vi "ActionVIOnLoad.vi"(8 "error in (no error)":errorcluster, 11 "Device Item Ref in":T1 format="%.0x") -> (0 "error out":errorcluster, 3 "Device Item Ref out":T1 format="%.0x")   [LabVIEW 2015, in "J1939 Addon System Explorer.lvlib"]
uses:
  J1939 Addon System Explorer.lvlib
  <vilib>/NI Veristand/Custom Device API/Custom Device Item Ref.ctl
  Shared/Types/XNET Settings.ctl
  Shared/Types/Monitor Settings.ctl
  Shared/Types/SPN Properties.ctl
  NationalInstruments.VeriStand.SystemDefinitionAPI
  Shared/SubVIs/Constants.vi
  <vilib>/NI Veristand/Custom Device API/Get Item Property (Variant).vi
  <vilib>/NI Veristand/Custom Device Tools/Custom Device Utility Library/NI VeriStand - Search for Item by GUID.vi
  <vilib>/NI Veristand/Custom Device API/Get Item Property (U16).vi
  <vilib>/NI Veristand/Custom Device API/Set Item Property (String).vi
  <vilib>/NI Veristand/Custom Device Tools/Custom Device Utility Library/NI VeriStand - Search for All Items by GUID.vi
  <vilib>/NI VeriStand/Custom Device API/Custom Device API.lvlib
  Shared/J1939 Addon Shared.lvlib
  <vilib>/NI VeriStand/Custom Device Tools/Custom Device Utility Library/Custom Device Utility Library.lvlib
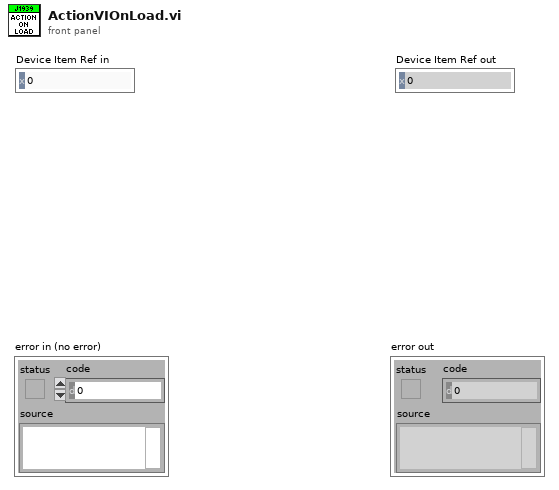
[diagram p1: front panel]
types:
  T1 = typedef "Custom Device API.lvlib/Custom Device Item Ref.ctl" = u64
  T2 = typedef "J1939 Addon Shared.lvlib/Monitor Settings.ctl" = cluster{"Address":u8, "Name":u64, "Include DA":bool}
  T3 = typedef "J1939 Addon Shared.lvlib/XNET Settings.ctl" = cluster{"Database":refnum<k21>, "Cluster":refnum<k21>, "Port":string, "Baud rate [Bd]":u32, "Termination":u32, "Incoming Decimation":u32, "Outgoing Decimation":u32}
  T4 = cluster{"XNET Database":refnum<k21>, "XNET Cluster":refnum<k21>, "CAN Port":string, "Baud rate [Bd]":u32, "J1939 Network Address":u8, "Name":u64, "Termination":u32}
  T5 = cluster{"XNET Database":refnum<k21>, "XNET Cluster":refnum<k21>, "CAN Port":string, "Baud rate [Bd]":u32, "J1939 Network Address":u8, "Name":u64, "Termination":u32, "Incoming Rate":u32, "Outcoming Rate":u32}
  T6 = cluster{"Database":refnum<k21>, "Cluster":refnum<k21>, "Port":string, "Baud rate [Bd]":u32, "Termination":u32, "Incoming Rate":u32, "Outcoming Rate":u32, "Write Decimation":u32}
  T7 = typedef "J1939 Addon Shared.lvlib/SPN Properties.ctl" = cluster{"Bytes":u32, "ScaleFac":dbl, "ScaleOff":dbl}
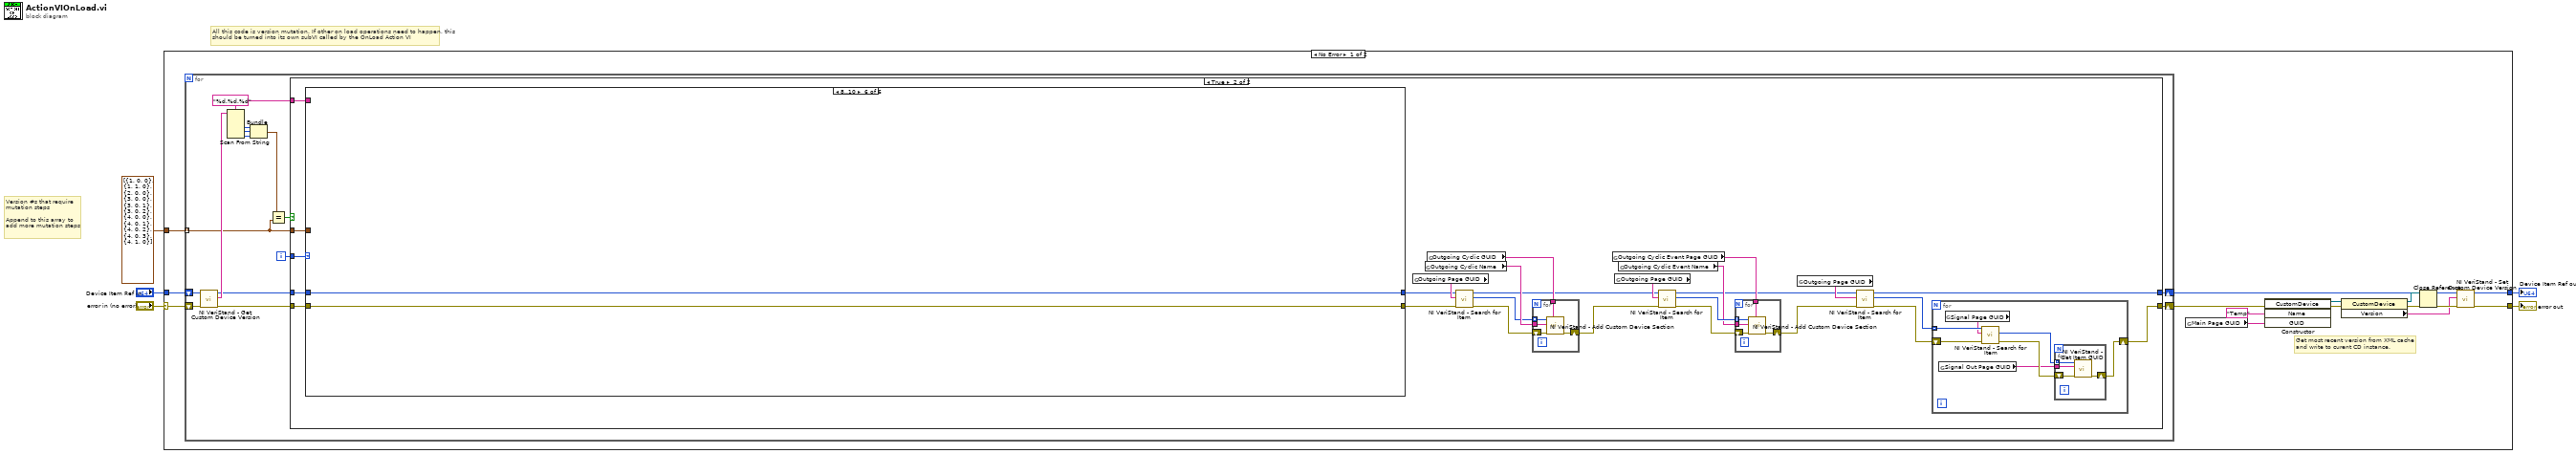
[diagram p0: block diagram]
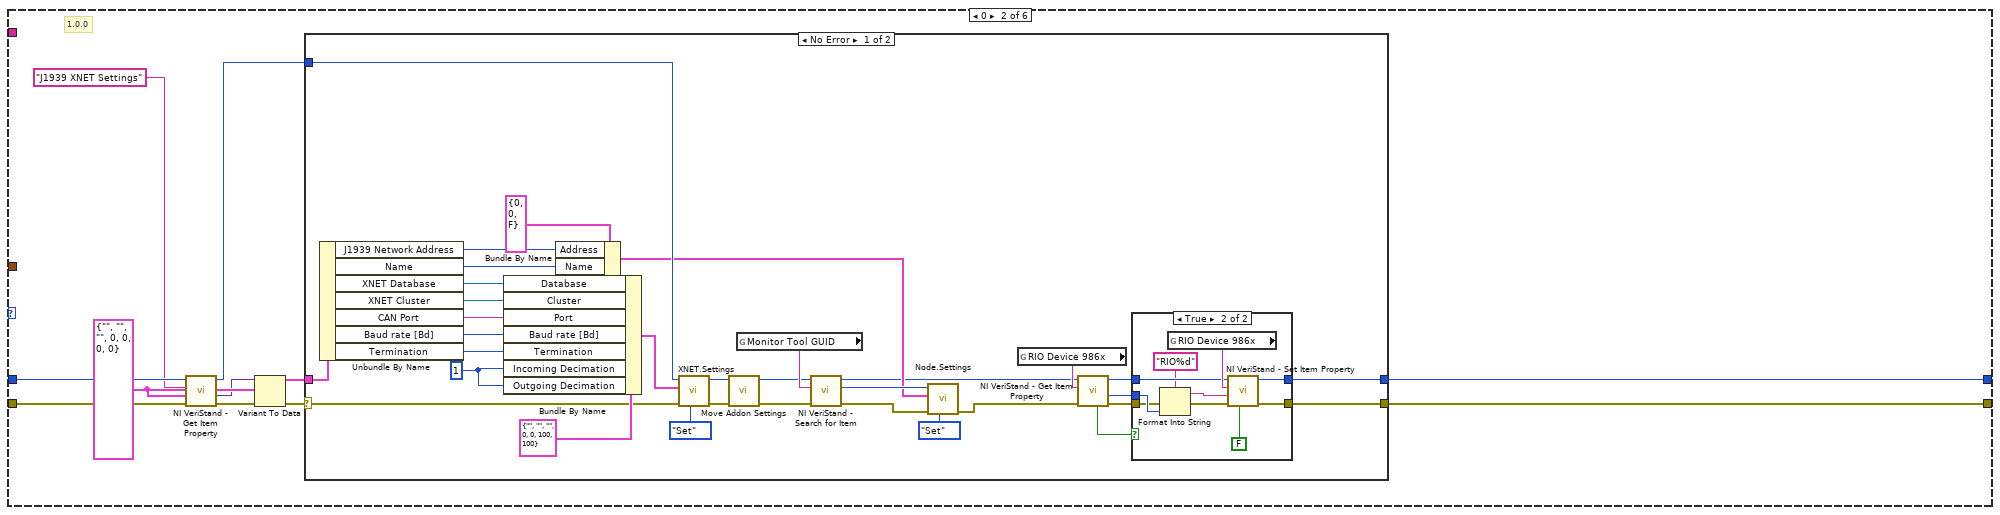
[diagram p4: hidden frame]
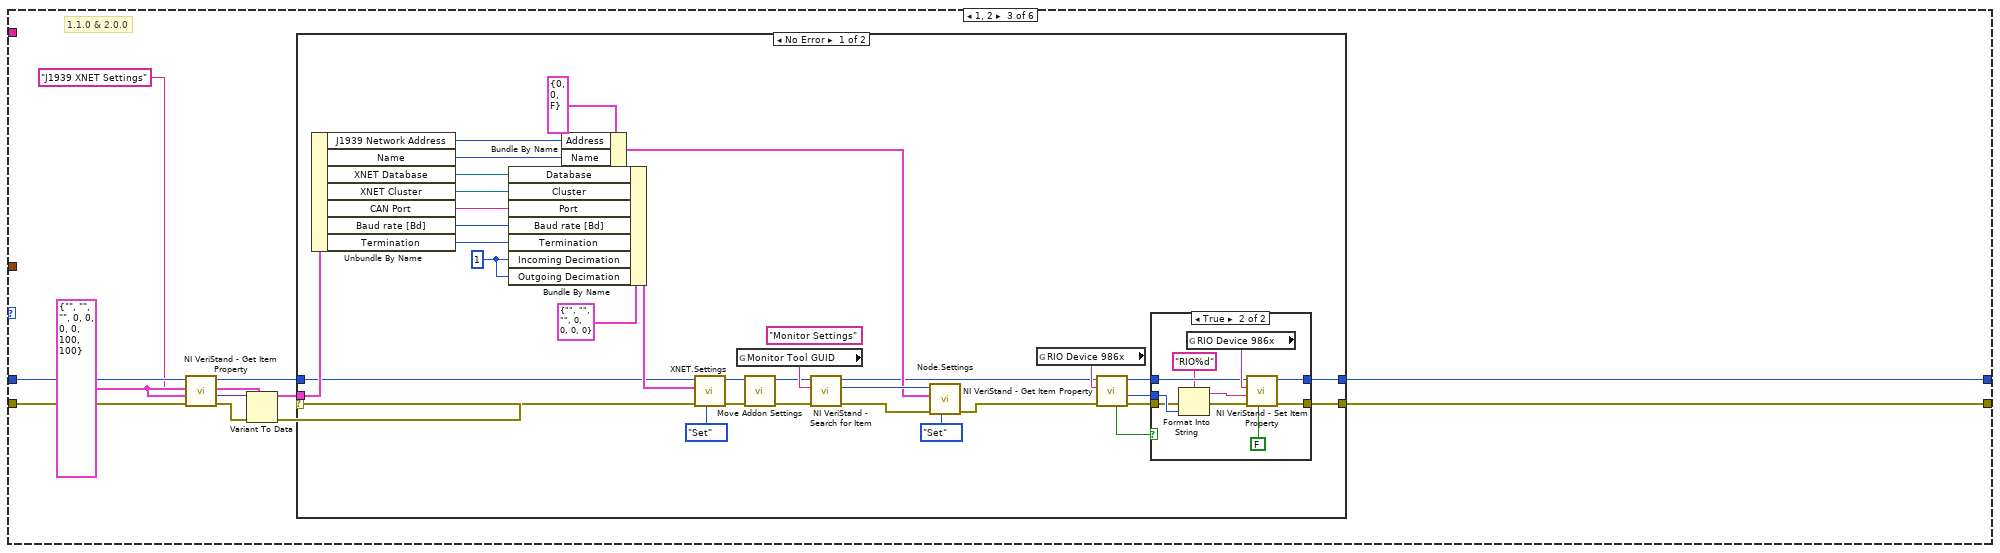
[diagram p7: hidden frame]
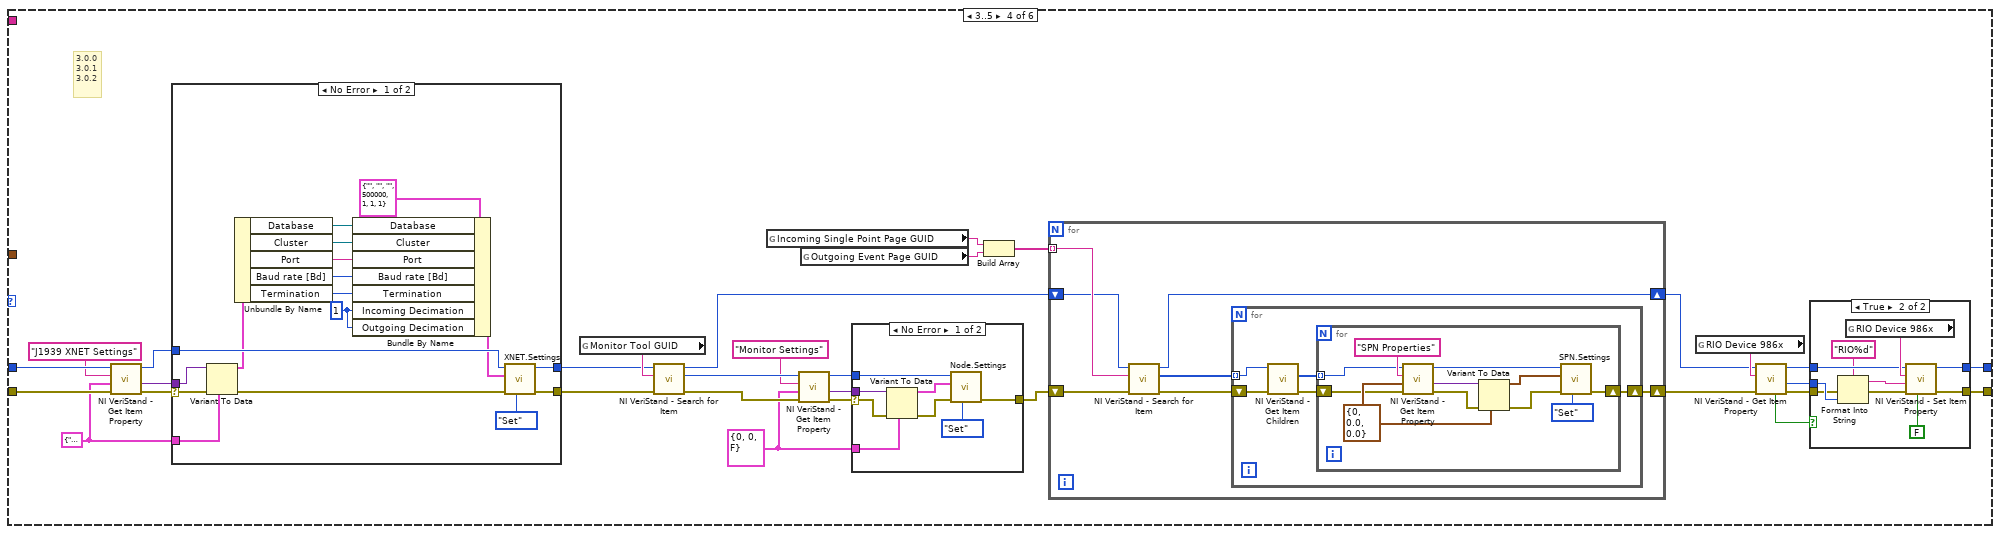
[diagram p10: hidden frame]
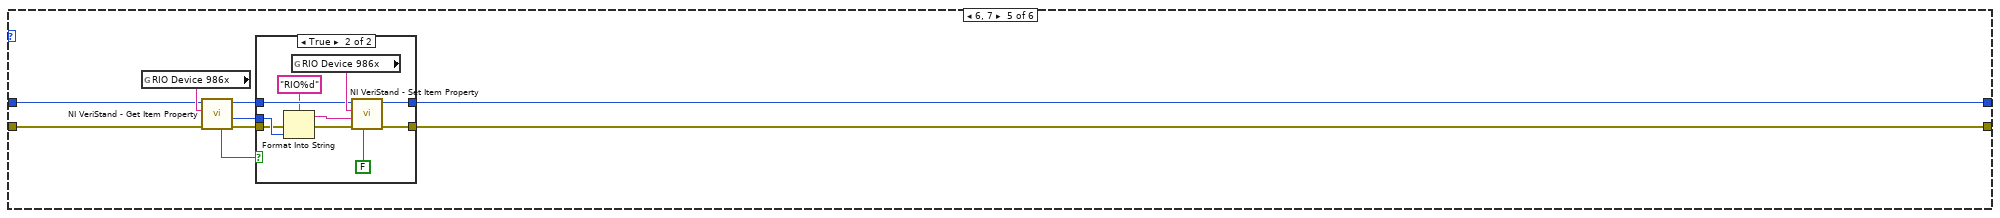
[diagram p14: hidden frame]
diagram:
  # "All this code is version mutation. If other on load operations need to happen, this should be turned into its own subVI called by the OnLoad Action VI"
  # "Version #s that require\nmutation steps\n\nAppend to this array to\nadd more mutation steps"
  n1 = case shown="No Error" "error in (no error)" {
    selector: "error in (no error)" -> [w19 w321]
    tunnel: [w11 w321] -> w1
    tunnel: "Device Item Ref in" -> [w18 w320]
    tunnel: [w10 w320] -> w2
    tunnel: cluster{i32, i32, i32}[] [{1, 0, 0}, {1, 1, 0}, {2, 0, 0}, {3, 0, 0}, {3, 0, 1}, {3, 0, 2}, {4, 0, 0}, {4, 0, 1}, {4, 0, 2}, {4, 0, 3}, {4, 1, 0}] -> [w20 _]
    frame No Error {
      # "Get most recent version from XML cache\nand write to curent CD instance."
      n2 = for {
        tunnel: w20 -> [w23] mode=indexing
        shift-right: [w28] -> w8
        shift-left: w19 -> [w33]
        shift-right: [w26] -> w9
        shift-left: w18 -> [w32]
        i -> [w25]
        w24 = "%d.%d.%d" ("format string")
        n3 = call <vilib>:"NI VeriStand - Get Custom Device Version.vi"("error in (no error)"=w33, "Device Ref in"=w32) -> ("error out"=w29:errorcluster, "Value"=w31:string, "Device Ref out"=w27:T1)  [unwired: 7 in]
        n4 = Scan From String(format string=w24, input string=w31) -> (output 1=w34:i32, output 2=w35:i32, output 3=w22:i32)  [unwired: 5 in, 3 out]
        n5 = Bundle(w34, w35, w22) -> (w21:cluster{i32, i32, i32})  [unwired: 1 in]
        n6 = Equal?(x=w21, y=w23) -> (x = y?=w30:bool)
        n7 = case shown="True" w30 {
          tunnel: w29 -> [w37 w63]
          tunnel: [w37 w38] -> w28
          tunnel: w27 -> [w36 w61]
          tunnel: [w36 w41] -> w26
          tunnel: w25 -> [_ w62]
          tunnel: w23 -> [_ w60]
          tunnel: w24 -> [_ w59]
          frame False {
          }
          frame True {
            n8 = case shown="8..10" w62 {
              tunnel: w63 -> [w81 w89 w148 w227 w295 w314]
              tunnel: [w81 w85 w144 w199 w293 w314] -> w53
              tunnel: [w80 w84 w143 w198 w292 w313] -> w52
              tunnel: w61 -> [w80 w88 w147 w228 w294 w313]
              tunnel: w60 -> [_ _ _ _ _ _]
              tunnel: w59 -> [_ _ _ _ _ _]
              frame Default {
              }
              frame 0 {
                w92 = T4 {"XNET Database"="", "XNET Cluster"="", "CAN Port"="", "Baud rate [Bd]"=0, "J1939 Network Address"=0, "Name"=0, "Termination"=0} ("J1939 XNET Settings")
                # "1.0.0"
                n9 = call-poly <vilib>:"NI VeriStand - Get Item Property.vi"("error in (no error)"=w89, "Default Value"=w92, "Property Name"="J1939 XNET Settings" ("J1939 XNET Settings"), "Item Ref in"=w88) -> ("error out"=w90:errorcluster, "Value"=w91:variant, "Item Ref out"=w86:T1)  [unwired: 4 in, 1 out]
                n10 = Variant To Data(error in=w90, type=w92, Variant=w91) -> (data=w87:T4, error out=w83:errorcluster)
                n11 = case shown="No Error" w83 {
                  selector: w83 -> [w118 w138]
                  tunnel: w87 -> [w125 _]
                  tunnel: w86 -> [w119 w139]
                  tunnel: [w97 w138] -> w85
                  tunnel: [w93 w139] -> w84
                  frame No Error {
                    w111 = u32 1 ("Incoming Rate")
                    n12 = Unbundle By Name(w125) -> ("J1939 Network Address"=w113:u8, "Name"=w114:u64, "XNET Database"=w123:refnum<k21>, "XNET Cluster"=w122:refnum<k21>, "CAN Port"=w121:string, "Baud rate [Bd]"=w120:u32, "Termination"=w116:u32)
                    n13 = Bundle By Name(cluster=T3 {"Database"="", "Cluster"="", "Port"="", "Baud rate [Bd]"=0, "Termination"=0, "Incoming Decimation"=100, "Outgoing Decimation"=100} ("J1939 XNET Settings"), "Database"=w123, "Cluster"=w122, "Port"=w121, "Baud rate [Bd]"=w120, "Termination"=w116, "Incoming Decimation"=w111, "Outgoing Decimation"=w111) -> (w105:T3)
                    n14 = Bundle By Name(cluster=T2 {"Address"=0, "Name"=0, "Include DA"=FALSE} ("J1939 Monitor Settings"), "Address"=w113, "Name"=w114) -> (w103:T2)
                    n15 = call "XNET.Settings.vi"("Action"=enum8{"Get", "Set"}."Set", "error in (no error)"=w118, "J1939 XNET Settings"=w105, "Parent Ref in"=w119) -> ("error out"=w107:errorcluster, "Item Ref out"=w109:T1)  [unwired: 5 in, 1 out]
                    n16 = call "Move Addon Settings.vi"("error in (no error)"=w107, "Section Ref in"=w109) -> ("error out"=w106:errorcluster, "Parent Ref out"=w108:T1)  [unwired: 8 in]
                    n17 = global read "Constants.vi" "Monitor Tool GUID"() -> (w117:string)
                    n18 = call-poly <vilib>:"NI VeriStand - Search for Item.vi"("error in"=w106, "Item GUID"=w117, "Section Ref in"=w108) -> ("error out"=w112:errorcluster, "Item Ref"=w110:T1, "Section Ref out"=w94:T1)  [unwired: 5 in, 1 out]
                    n19 = call "Node.Settings.vi"("Action"=enum8{"Get", "Set"}."Set", "error in (no error)"=w112, "Node.Settings"=w103, "Item Ref in"=w110) -> ("error out"=w100:errorcluster)  [unwired: 5 in, 2 out]
                    n20 = global read "Constants.vi" "RIO Device 986x"() -> (w101:string)
                    n21 = call-poly <vilib>:"NI VeriStand - Get Item Property.vi"("error in (no error)"=w100, "Property Name"=w101, "Item Ref in"=w94) -> ("error out"=w98:errorcluster, "Value"=w95:u16, "Item Ref out"=w99:T1, "Found?"=w96:bool)  [unwired: 5 in]
                    n22 = case shown="True" w96 {
                      tunnel: w99 -> [w126 w136]
                      tunnel: w98 -> [w127 w132]
                      tunnel: [w127 w135] -> w97
                      tunnel: w95 -> [_ w133]
                      tunnel: [w126 w129] -> w93
                      frame False {
                      }
                      frame True {
                        n23 = Format Into String(format string="RIO%d", error in=w132, w133) -> (resulting string=w128:string, error out=w131:errorcluster)  [unwired: 1 in]
                        n24 = global read "Constants.vi" "RIO Device 986x"() -> (w137:string)
                        n25 = call-poly <vilib>:"NI VeriStand - Set Item Property.vi"("Binary String (T)"=FALSE ("Replaced"), "error in (no error)"=w131, "Value"=w128, "Property Name"=w137, "Item Ref in"=w136) -> ("error out"=w135:errorcluster, "Item Ref out"=w129:T1)  [unwired: 4 in, 1 out]
                      }
                    }
                  }
                  frame Error {
                  }
                }
              }
              frame 1, 2 {
                w141 = T5 {"XNET Database"="", "XNET Cluster"="", "CAN Port"="", "Baud rate [Bd]"=0, "J1939 Network Address"=0, "Name"=0, "Termination"=0, "Incoming Rate"=100, "Outcoming Rate"=100} ("J1939 XNET Settings")
                # "1.1.0 & 2.0.0"
                n26 = call-poly <vilib>:"NI VeriStand - Get Item Property.vi"("error in (no error)"=w148, "Default Value"=w141, "Property Name"="J1939 XNET Settings" ("J1939 XNET Settings"), "Item Ref in"=w147) -> ("error out"=w149:errorcluster, "Value"=w150:variant, "Item Ref out"=w145:T1)  [unwired: 4 in, 1 out]
                n27 = Variant To Data(error in=w149, type=w141, Variant=w150) -> (data=w146:T5, error out=w142:errorcluster)
                n28 = case shown="No Error" w142 {
                  selector: w142 -> [w162 w196]
                  tunnel: w146 -> [w183 _]
                  tunnel: w145 -> [w161 w197]
                  tunnel: [w153 w196] -> w144
                  tunnel: [w151 w197] -> w143
                  frame No Error {
                    w160 = u32 1 ("Incoming Decimation")
                    (unwired) "Monitor Settings" ("J1939 Monitor Settings")
                    n29 = Unbundle By Name(w183) -> ("J1939 Network Address"=w173:u8, "Name"=w174:u64, "XNET Database"=w181:refnum<k21>, "XNET Cluster"=w180:refnum<k21>, "CAN Port"=w179:string, "Baud rate [Bd]"=w178:u32, "Termination"=w176:u32)
                    n30 = Bundle By Name(cluster=T3 {"Database"="", "Cluster"="", "Port"="", "Baud rate [Bd]"=0, "Termination"=0, "Incoming Decimation"=0, "Outgoing Decimation"=0} ("J1939 XNET Settings"), "Database"=w181, "Cluster"=w180, "Port"=w179, "Baud rate [Bd]"=w178, "Termination"=w176, "Incoming Decimation"=w160, "Outgoing Decimation"=w160) -> (w166:T3)
                    n31 = Bundle By Name(cluster=T2 {"Address"=0, "Name"=0, "Include DA"=FALSE} ("J1939 Monitor Settings"), "Address"=w173, "Name"=w174) -> (w165:T2)
                    n32 = call "XNET.Settings.vi"("Action"=enum8{"Get", "Set"}."Set", "error in (no error)"=w162, "J1939 XNET Settings"=w166, "Parent Ref in"=w161) -> ("error out"=w168:errorcluster, "Item Ref out"=w170:T1)  [unwired: 5 in, 1 out]
                    n33 = global read "Constants.vi" "Monitor Tool GUID"() -> (w177:string)
                    n34 = call "Move Addon Settings.vi"("error in (no error)"=w168, "Section Ref in"=w170) -> ("error out"=w167:errorcluster, "Parent Ref out"=w169:T1)  [unwired: 8 in]
                    n35 = call-poly <vilib>:"NI VeriStand - Search for Item.vi"("error in"=w167, "Item GUID"=w177, "Section Ref in"=w169) -> ("error out"=w172:errorcluster, "Item Ref"=w171:T1, "Section Ref out"=w152:T1)  [unwired: 5 in, 1 out]
                    n36 = call "Node.Settings.vi"("Action"=enum8{"Get", "Set"}."Set", "error in (no error)"=w172, "Node.Settings"=w165, "Item Ref in"=w171) -> ("error out"=w154:errorcluster)  [unwired: 5 in, 2 out]
                    n37 = global read "Constants.vi" "RIO Device 986x"() -> (w159:string)
                    n38 = call-poly <vilib>:"NI VeriStand - Get Item Property.vi"("error in (no error)"=w154, "Property Name"=w159, "Item Ref in"=w152) -> ("error out"=w157:errorcluster, "Value"=w155:u16, "Item Ref out"=w158:T1, "Found?"=w156:bool)  [unwired: 5 in]
                    n39 = case shown="True" w156 {
                      tunnel: w158 -> [w184 w194]
                      tunnel: w157 -> [w185 w190]
                      tunnel: [w185 w193] -> w153
                      tunnel: w155 -> [_ w191]
                      tunnel: [w184 w187] -> w151
                      frame False {
                      }
                      frame True {
                        n40 = Format Into String(format string="RIO%d", error in=w190, w191) -> (resulting string=w186:string, error out=w189:errorcluster)  [unwired: 1 in]
                        n41 = global read "Constants.vi" "RIO Device 986x"() -> (w195:string)
                        n42 = call-poly <vilib>:"NI VeriStand - Set Item Property.vi"("Binary String (T)"=FALSE ("Replaced"), "error in (no error)"=w189, "Value"=w186, "Property Name"=w195, "Item Ref in"=w194) -> ("error out"=w193:errorcluster, "Item Ref out"=w187:T1)  [unwired: 4 in, 1 out]
                      }
                    }
                  }
                  frame Error {
                  }
                }
              }
              frame 3..5 {
                w212 = T2 {"Address"=0, "Name"=0, "Include DA"=FALSE} ("J1939 Monitor Settings")
                w223 = T6 {"Database"="", "Cluster"="", "Port"="", "Baud rate [Bd]"=0, "Termination"=0, "Incoming Rate"=0, "Outcoming Rate"=0, "Write Decimation"=0} ("J1939 XNET Settings")
                # "3.0.0\n3.0.1\n3.0.2"
                n43 = call-poly <vilib>:"NI VeriStand - Get Item Property.vi"("error in (no error)"=w227, "Default Value"=w223, "Property Name"="J1939 XNET Settings" ("J1939 XNET Settings"), "Item Ref in"=w228) -> ("error out"=w225:errorcluster, "Value"=w224:variant, "Item Ref out"=w222:T1)  [unwired: 4 in, 1 out]
                n44 = case shown="No Error" w225 {
                  selector: w225 -> [w257 w259]
                  tunnel: w224 -> [w256 _]
                  tunnel: w223 -> [w255 _]
                  tunnel: w222 -> [w252 w258]
                  tunnel: [w251 w258] -> w219
                  tunnel: [w250 w259] -> w220
                  frame No Error {
                    w241 = u32 1 ("Incoming Decimation")
                    n45 = Variant To Data(error in=w257, type=w255, Variant=w256) -> (data=w247:T6, error out=w253:errorcluster)
                    n46 = Unbundle By Name(w247) -> ("Database"=w246:refnum<k21>, "Cluster"=w242:refnum<k21>, "Port"=w243:string, "Baud rate [Bd]"=w244:u32, "Termination"=w245:u32)
                    n47 = Bundle By Name(cluster=T3 {"Database"="", "Cluster"="", "Port"="", "Baud rate [Bd]"=500000, "Termination"=1, "Incoming Decimation"=1, "Outgoing Decimation"=1} ("J1939 XNET Settings"), "Database"=w246, "Cluster"=w242, "Port"=w243, "Baud rate [Bd]"=w244, "Termination"=w245, "Incoming Decimation"=w241, "Outgoing Decimation"=w241) -> (w248:T3)
                    n48 = call "XNET.Settings.vi"("Action"=enum8{"Get", "Set"}."Set", "error in (no error)"=w253, "J1939 XNET Settings"=w248, "Parent Ref in"=w252) -> ("error out"=w250:errorcluster, "Item Ref out"=w251:T1)  [unwired: 5 in, 1 out]
                  }
                  frame Error {
                  }
                }
                n49 = global read "Constants.vi" "Monitor Tool GUID"() -> (w221:string)
                n50 = call-poly <vilib>:"NI VeriStand - Search for Item.vi"("error in"=w220, "Item GUID"=w221, "Section Ref in"=w219) -> ("error out"=w218:errorcluster, "Item Ref"=w217:T1, "Section Ref out"=w207:T1)  [unwired: 5 in, 1 out]
                n51 = global read "Constants.vi" "Incoming Single Point Page GUID"() -> (w210:string)
                n52 = call-poly <vilib>:"NI VeriStand - Get Item Property.vi"("error in (no error)"=w218, "Default Value"=w212, "Property Name"="Monitor Settings" ("J1939 Monitor Settings"), "Item Ref in"=w217) -> ("error out"=w213:errorcluster, "Value"=w214:variant, "Item Ref out"=w215:T1)  [unwired: 4 in, 1 out]
                n53 = global read "Constants.vi" "Outgoing Event Page GUID"() -> (w209:string)
                n54 = case shown="No Error" w213 {
                  selector: w213 -> [w290 w291]
                  tunnel: w214 -> [w289 _]
                  tunnel: w212 -> [w288 _]
                  tunnel: w215 -> [w285 _]
                  tunnel: [w284 w291] -> w208
                  frame No Error {
                    n55 = Variant To Data(error in=w290, type=w288, Variant=w289) -> (data=w283:T2, error out=w286:errorcluster)
                    n56 = call "Node.Settings.vi"("Action"=enum8{"Get", "Set"}."Set", "error in (no error)"=w286, "Node.Settings"=w283, "Item Ref in"=w285) -> ("error out"=w284:errorcluster)  [unwired: 5 in, 2 out]
                  }
                  frame Error {
                  }
                }
                n57 = Build Array(w210, w209) -> (w211:string[])
                n58 = for {
                  tunnel: w211 -> [w266] mode=indexing
                  shift-right: [w263] -> w201
                  shift-left: w208 -> [w262]
                  shift-right: [w261] -> w200
                  shift-left: w207 -> [w260]
                  n59 = call-poly <vilib>:"NI VeriStand - Search for Item.vi"("error in"=w262, "Item GUID"=w266, "Section Ref in"=w260) -> ("error out"=w264:errorcluster, "Item Refs"=w265:T1[], "Section Ref out"=w261:T1)  [unwired: 5 in, 1 out]
                  n60 = for {
                    tunnel: w265 -> [w270] mode=indexing
                    shift-right: [w267] -> w263
                    shift-left: w264 -> [w271]
                    n61 = call <vilib>:"NI VeriStand - Get Item Children.vi"("error in (no error)"=w271, "Item Ref in"=w270) -> ("error out"=w268:errorcluster, "Child Refs"=w269:T1[])  [unwired: 6 in, 2 out]
                    n62 = for {
                      tunnel: w269 -> [w277] mode=indexing
                      shift-right: [w273] -> w267
                      shift-left: w268 -> [w278]
                      w281 = T7 {"Bytes"=0, "ScaleFac"=0.0, "ScaleOff"=0.0} ("cluster")
                      n63 = call-poly <vilib>:"NI VeriStand - Get Item Property.vi"("error in (no error)"=w278, "Default Value"=w281, "Property Name"="SPN Properties" ("SPN Properties"), "Item Ref in"=w277) -> ("error out"=w280:errorcluster, "Value"=w279:variant, "Item Ref out"=w276:T1)  [unwired: 4 in, 1 out]
                      n64 = Variant To Data(error in=w280, type=w281, Variant=w279) -> (data=w275:T7, error out=w274:errorcluster)
                      n65 = call "SPN.Settings.vi"("Action"=enum8{"Get", "Set"}."Set", "error in (no error)"=w274, "SPN.Settings"=w275, "Item Ref in"=w276) -> ("error out"=w273:errorcluster)  [unwired: 5 in, 2 out]
                    }
                  }
                }
                n66 = global read "Constants.vi" "RIO Device 986x"() -> (w206:string)
                n67 = call-poly <vilib>:"NI VeriStand - Get Item Property.vi"("error in (no error)"=w201, "Property Name"=w206, "Item Ref in"=w200) -> ("error out"=w204:errorcluster, "Value"=w202:u16, "Item Ref out"=w205:T1, "Found?"=w203:bool)  [unwired: 5 in]
                n68 = case shown="True" w203 {
                  tunnel: w205 -> [w229 w239]
                  tunnel: w204 -> [w230 w235]
                  tunnel: [w230 w238] -> w199
                  tunnel: w202 -> [_ w236]
                  tunnel: [w229 w232] -> w198
                  frame False {
                  }
                  frame True {
                    n69 = Format Into String(format string="RIO%d", error in=w235, w236) -> (resulting string=w231:string, error out=w234:errorcluster)  [unwired: 1 in]
                    n70 = global read "Constants.vi" "RIO Device 986x"() -> (w240:string)
                    n71 = call-poly <vilib>:"NI VeriStand - Set Item Property.vi"("Binary String (T)"=FALSE ("Replaced"), "error in (no error)"=w234, "Value"=w231, "Property Name"=w240, "Item Ref in"=w239) -> ("error out"=w238:errorcluster, "Item Ref out"=w232:T1)  [unwired: 4 in, 1 out]
                  }
                }
              }
              frame 6, 7 {
                n72 = global read "Constants.vi" "RIO Device 986x"() -> (w300:string)
                n73 = call-poly <vilib>:"NI VeriStand - Get Item Property.vi"("error in (no error)"=w295, "Property Name"=w300, "Item Ref in"=w294) -> ("error out"=w298:errorcluster, "Value"=w296:u16, "Item Ref out"=w299:T1, "Found?"=w297:bool)  [unwired: 5 in]
                n74 = case shown="True" w297 {
                  tunnel: w299 -> [w301 w311]
                  tunnel: w298 -> [w302 w307]
                  tunnel: [w302 w310] -> w293
                  tunnel: w296 -> [_ w308]
                  tunnel: [w301 w304] -> w292
                  frame False {
                  }
                  frame True {
                    n75 = Format Into String(format string="RIO%d", error in=w307, w308) -> (resulting string=w303:string, error out=w306:errorcluster)  [unwired: 1 in]
                    n76 = global read "Constants.vi" "RIO Device 986x"() -> (w312:string)
                    n77 = call-poly <vilib>:"NI VeriStand - Set Item Property.vi"("Binary String (T)"=FALSE ("Replaced"), "error in (no error)"=w306, "Value"=w303, "Property Name"=w312, "Item Ref in"=w311) -> ("error out"=w310:errorcluster, "Item Ref out"=w304:T1)  [unwired: 4 in, 1 out]
                  }
                }
              }
              frame 8..10 {
              }
            }
            n78 = global read "Constants.vi" "Outgoing Page GUID"() -> (w58:string)
            n79 = global read "Constants.vi" "Outgoing Cyclic Name"() -> (w56:string)
            n80 = global read "Constants.vi" "Outgoing Cyclic GUID"() -> (w57:string)
            n81 = call-poly <vilib>:"NI VeriStand - Search for Item.vi"("error in"=w53, "Item GUID"=w58, "Section Ref in"=w52) -> ("error out"=w54:errorcluster, "Item Refs"=w55:T1[], "Section Ref out"=w45:T1)  [unwired: 5 in, 1 out]
            n82 = for {
              tunnel: w57 -> [w319]
              tunnel: w56 -> [w318]
              tunnel: w55 -> [w317] mode=indexing
              shift-right: [w315] -> w46
              shift-left: w54 -> [w316]
              n83 = call <vilib>:"NI VeriStand - Add Custom Device Section.vi"("GUID (Default Section)"=w319, "error in (no error)"=w316, "Section Name"=w318, "Parent Ref in"=w317) -> ("error out"=w315:errorcluster)  [unwired: 4 in, 3 out]
            }
            n84 = global read "Constants.vi" "Outgoing Cyclic Event Page GUID"() -> (w48:string)
            n85 = global read "Constants.vi" "Outgoing Page GUID"() -> (w47:string)
            n86 = global read "Constants.vi" "Outgoing Cyclic Event Name"() -> (w49:string)
            n87 = call-poly <vilib>:"NI VeriStand - Search for Item.vi"("error in"=w46, "Item GUID"=w47, "Section Ref in"=w45) -> ("error out"=w51:errorcluster, "Item Refs"=w50:T1[], "Section Ref out"=w42:T1)  [unwired: 5 in, 1 out]
            n88 = for {
              tunnel: w48 -> [w79]
              tunnel: w49 -> [w78]
              tunnel: w50 -> [w77] mode=indexing
              shift-right: [w75] -> w43
              shift-left: w51 -> [w76]
              n89 = call <vilib>:"NI VeriStand - Add Custom Device Section.vi"("GUID (Default Section)"=w79, "error in (no error)"=w76, "Section Name"=w78, "Parent Ref in"=w77) -> ("error out"=w75:errorcluster)  [unwired: 4 in, 3 out]
            }
            n90 = global read "Constants.vi" "Outgoing Page GUID"() -> (w44:string)
            n91 = call-poly <vilib>:"NI VeriStand - Search for Item.vi"("error in"=w43, "Item GUID"=w44, "Section Ref in"=w42) -> ("error out"=w39:errorcluster, "Item Refs"=w40:T1[], "Section Ref out"=w41:T1)  [unwired: 5 in, 1 out]
            n92 = for {
              tunnel: w40 -> [w70] mode=indexing
              shift-right: [w65] -> w38
              shift-left: w39 -> [w68]
              n93 = global read "Constants.vi" "Signal Out Page GUID"() -> (w64:string)
              n94 = global read "Constants.vi" "Signal Page GUID"() -> (w69:string)
              n95 = call-poly <vilib>:"NI VeriStand - Search for Item.vi"("error in"=w68, "Item GUID"=w69, "Section Ref in"=w70) -> ("error out"=w66:errorcluster, "Item Refs"=w67:T1[])  [unwired: 5 in, 2 out]
              n96 = for {
                tunnel: w67 -> [w74] mode=indexing
                shift-right: [w72] -> w65
                shift-left: w66 -> [w73]
                tunnel: w64 -> [w71]
                n97 = call <vilib>:"NI VeriStand - Set Item GUID.vi"("error in (no error)"=w73, "GUID"=w71, "Item Ref in"=w74) -> ("error out"=w72:errorcluster)  [unwired: 7 in, 1 out]
              }
            }
          }
        }
      }
      n98 = global read "Constants.vi" "Main Page GUID"() -> (w6:string)
      n99 = constructor class="CustomDevice"(error in=w8, "Name"="Temp", "GUID"=w6) -> (reference out=w17:refnum<k24>, error out=w16:errorcluster)  [unwired: 2 in, 3 out]
      n100 = property class="CustomDevice"(reference=w17, error in=w16) -> (reference out=w14:refnum<k24>, error out=w15:errorcluster, "Version"=w12:string)
      n101 = Close Reference(reference=w14, error in (no error)=w15) -> (error out=w13:errorcluster)
      n102 = call <vilib>:"NI VeriStand - Set Custom Device Version.vi"("error in (no error)"=w13, "Value"=w12, "Device Ref in"=w9) -> ("error out"=w11:errorcluster, "Device Ref out"=w10:T1)  [unwired: 7 in]
    }
    frame Error {
    }
  }
  "error out" <- w1
  "Device Item Ref out" <- w2
